vi "Update-filter-file-labels.vi"(8 "error in":errorcluster, 11 "Active filter array in":T1[](array[typedef])) -> (0 "error IO":errorcluster, 2 "Report labels":string[](array[string]))   [LabVIEW 2013, in "CameraVision.lvlib" / "CV-Filter.lvclass"]
uses:
  CV-Filter.lvclass
  Filter-settings.ctl
  Filter-characteristic.ctl
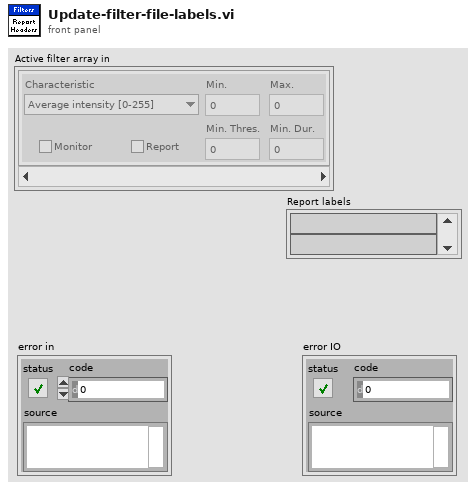
[diagram p1: front panel]
types:
  T1 = typedef "CameraVision.lvlib/CV-Filter.lvclass/Filter-settings.ctl" = cluster{"Characteristic":T2, "Monitor":bool, "Min.":dbl, "Max.":dbl, "Min. Thres.":dbl, "Min. Dur.":u16, "Report":bool}
  T2 = typedef "CameraVision.lvlib/CV-Filter.lvclass/Filter-characteristic.ctl" = enum16{"Average intensity [0-255]", "Peak intensity [0-255]", "Melt-pool size [mm²]", "Melt-pool aspect ratio []", "Melt-pool fragments []", "Melt-pool position X [pixel]", "Melt-pool position Y [pixel]", "Average temperature [°C]", "Max. temperature [°C]", "Min. temperature [°C]", "Std. dev. temperature [°C]"}
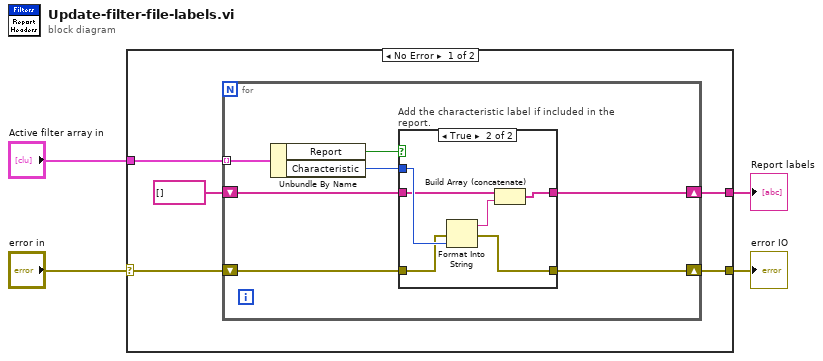
[diagram p0: block diagram]
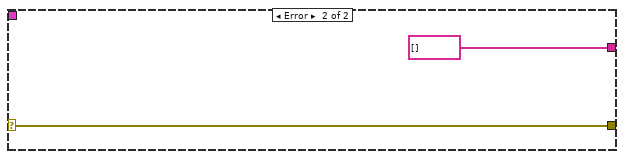
[diagram p3: hidden frame]
diagram:
  n1 = case shown="No Error" "error in" {
    selector: "error in" -> [w5 w26]
    tunnel: [w9 w26] -> w4
    tunnel: [w8 string[] []] -> w3
    tunnel: "Active filter array in" -> [w6 _]
    frame No Error {
      n2 = for {
        tunnel: w6 -> [w12] mode=indexing
        shift-right: [w15] -> w8
        shift-left: string[] [] -> [w16]
        shift-right: [w13] -> w9
        shift-left: w5 -> [w14]
        n3 = Unbundle By Name(w12) -> ("Report"=w10:bool, "Characteristic"=w11:T2)
        n4 = case "Add the characteristic label if included in the report." shown="True" w10 {
          tunnel: w16 -> [w18 w22]
          tunnel: w11 -> [_ w24]
          tunnel: [w18 w21] -> w15
          tunnel: w14 -> [w17 w20]
          tunnel: [w17 w19] -> w13
          frame False {
          }
          frame True {
            n5 = Format Into String(error in=w20, w24) -> (resulting string=w23:string, error out=w19:errorcluster)  [unwired: 2 in]
            n6 = Build Array (concatenate)(w22, w23) -> (w21:string[])
          }
        }
      }
    }
    frame Error {
    }
  }
  "error IO" <- w4
  "Report labels" <- w3
